vi "CreateSystemEvent_8532.vi"(8 "error in (no error)":errorcluster) -> (0 "error out":errorcluster, 3 "hEvent":i32)   [LabVIEW 2009]
uses:
  PCI8532_32.dll
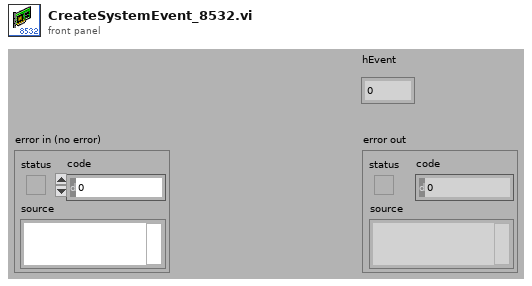
[diagram p1: front panel]
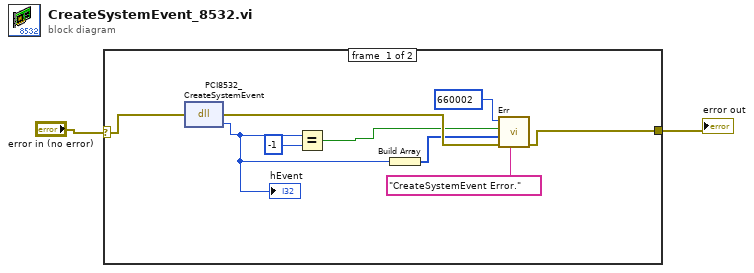
[diagram p0: block diagram]
diagram:
  n1 = case shown="无错误" "error in (no error)" {
    selector: "error in (no error)" -> [w11 w12]
    tunnel: [w8 w12] -> w1
    frame #0 {
      n2 = dll-call lib="PCI8532_32.dll" fn="PCI8532_CreateSystemEvent" label="CreateSystemEvent"(error in=w11) -> (error out=w9:errorcluster, "hEvent"=w4:i32)  [unwired: 2 in, 1 out]
      "hEvent" <- w4
      n3 = Equal?(x=w4, y=-1) -> (x = y?=w7:bool)
      n4 = Build Array(w4) -> (w5:i32[])
      n5 = call "Err.vi"("source"="CreateSystemEvent Error.", "error in (no error)"=w9, "Par"=w5, "error?"=w7, "code"=660002) -> ("error out"=w8:errorcluster)  [unwired: 6 out]
    }
    frame #1 {
    }
  }
  "error out" <- w1
